vi "Launch_Server.vi"(7 "port":u16=6379, 8 "error in":errorcluster, 10 "working directory":path, 11 "host":string="localhost") -> (0 "error out":errorcluster, 2 "Server Alive ?":bool)   [LabVIEW 2020]
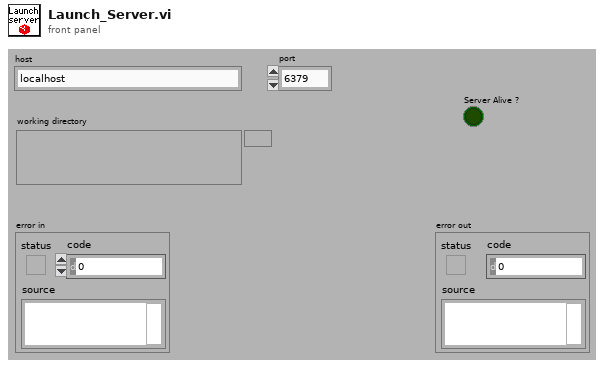
[diagram p1: front panel]
types:
  T1 = enum16{"None", "Error", "Status", "Nil", "Integer", "String", "Multibulk"}
  T2 = cluster{"integer":i64, "string":string, "multibulk":variant[]}
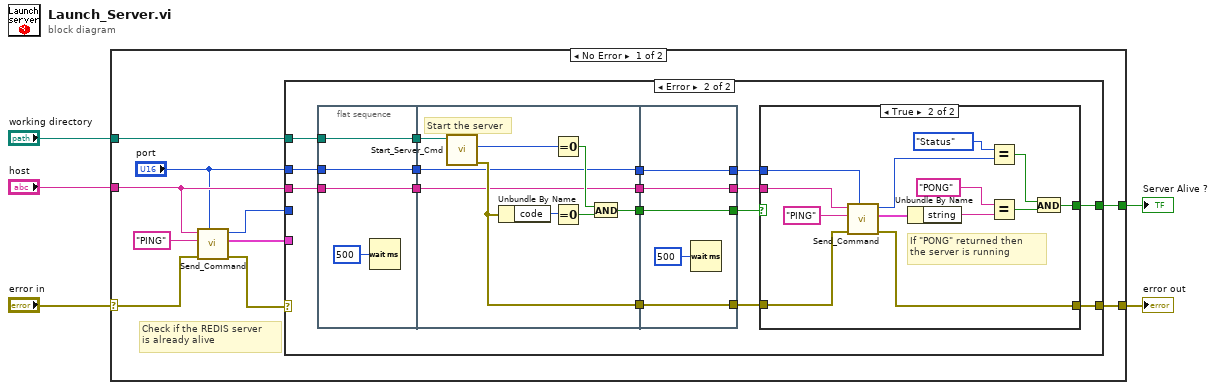
[diagram p0: block diagram]
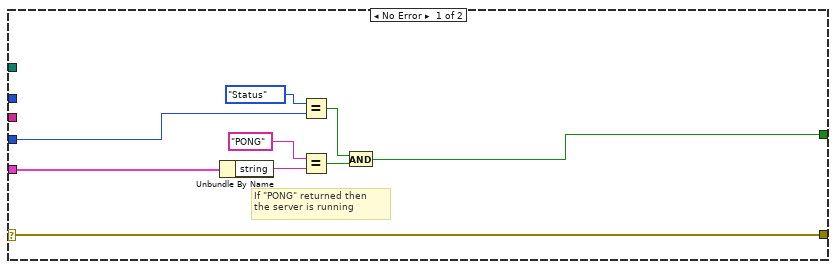
[diagram p2: hidden frame]
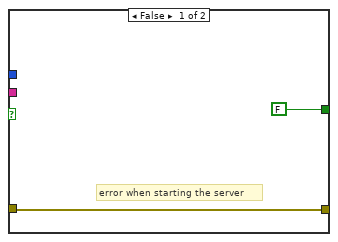
[diagram p3: hidden frame]
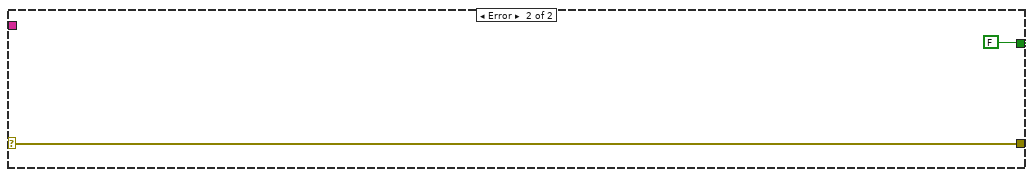
[diagram p4: hidden frame]
diagram:
  n1 = case shown="No Error" "error in" {
    selector: "error in" -> [w14 w75]
    tunnel: "host" -> [w7 _]
    tunnel: [w10 w75] -> w3
    tunnel: "working directory" -> [w9 _]
    tunnel: [w8 FALSE] -> w1
    frame No Error {
      # "Check if the REDIS server\nis already alive"
      n2 = call "Send_Command.vi"("port"="port", "error in"=w14, "command"="PING", "host"=w7) -> ("error out"=w13:errorcluster, "reply"=w12:T2, "type"=w11:T1)  [unwired: 4 in, 1 out]
      n3 = case shown="Error" w13 {
        selector: w13 -> [w17 _]
        tunnel: w12 -> [w22 _]
        tunnel: w11 -> [w24 _]
        tunnel: [w17 w36] -> w10
        tunnel: w9 -> [_ w40]
        tunnel: [w16 w38] -> w8
        tunnel: w7 -> [_ w28]
        tunnel: "port" -> [_ w32]
        frame No Error {
          # "If \"PONG\" returned then\nthe server is running"
          n4 = Unbundle By Name(w22) -> ("string"=w21:string)
          n5 = Equal?(x=T1."Status" ("type"), y=w24) -> (x = y?=w18:bool)
          n6 = Equal?(x="PONG", y=w21) -> (x = y?=w19:bool)
          n7 = And(x=w18, y=w19) -> (x .and. y?=w16:bool)
        }
        frame Error {
          n8 = flat-sequence {
            tunnel: w40 -> [w44]
            tunnel: [w44] -> w35
            tunnel: w32 -> [w43]
            tunnel: [w43] -> w31
            tunnel: w28 -> [w42]
            tunnel: [w42] -> w27
            tunnel: w35 -> [w49]
            tunnel: [w48] -> w34
            tunnel: [w47] -> w33
            tunnel: w31 -> [w46]
            tunnel: [w46] -> w30
            tunnel: w27 -> [w45]
            tunnel: [w45] -> w26
            tunnel: [w57] -> w37
            tunnel: [w58] -> w39
            tunnel: w34 -> [w58]
            tunnel: w33 -> [w57]
            tunnel: w30 -> [w56]
            tunnel: [w56] -> w29
            tunnel: w26 -> [w55]
            tunnel: [w55] -> w25
            frame #0 {
              n9 = Wait (ms)(milliseconds to wait=u32 500) -> ()  [unwired: 1 out]
            }
            frame #1 {
              # "Start the server"
              n10 = call "Start_Server_Cmd.vi"("working directory"=w49) -> ("error out"=w47:errorcluster, "return code"=w50:i32)  [unwired: 9 in]
              n11 = Unbundle By Name(w47) -> ("code"=w51:i32)
              n12 = Equal To 0?(x=w50) -> (x = 0?=w53:bool)
              n13 = Equal To 0?(x=w51) -> (x = 0?=w52:bool)
              n14 = And(x=w53, y=w52) -> (x .and. y?=w48:bool)
            }
            frame #2 {
              n15 = Wait (ms)(milliseconds to wait=u32 500) -> ()  [unwired: 1 out]
            }
          }
          n16 = case shown="True" w39 {
            tunnel: w25 -> [_ w65]
            tunnel: w29 -> [_ w64]
            tunnel: [FALSE w63] -> w38
            tunnel: w37 -> [w59 w62]
            tunnel: [w59 w61] -> w36
            frame False {
              # "error when starting the server"
            }
            frame True {
              # "If \"PONG\" returned then\nthe server is running"
              n17 = call "Send_Command.vi"("port"=w64, "error in"=w62, "command"="PING", "host"=w65) -> ("error out"=w61:errorcluster, "reply"=w72:T2, "type"=w73:T1)  [unwired: 4 in, 1 out]
              n18 = Unbundle By Name(w72) -> ("string"=w70:string)
              n19 = Equal?(x=T1."Status" ("type"), y=w73) -> (x = y?=w67:bool)
              n20 = Equal?(x="PONG", y=w70) -> (x = y?=w68:bool)
              n21 = And(x=w67, y=w68) -> (x .and. y?=w63:bool)
            }
          }
        }
      }
    }
    frame Error {
    }
  }
  "error out" <- w3
  "Server Alive ?" <- w1
